vi "G#Object_GetAttributeValue.vi"(0 "reference in":refnum<class "G#Object.lvclass">, 1 "object attributes (T)":bool=TRUE, 2 "class attributes (F)":bool, 5 "error in (no error)":errorcluster) -> (14 "reference out":refnum<class "G#Object.lvclass">, 15 "attributes":variant[](array[variant]), 16 "class attributes":variant[](array[variant]), 17 "valid object":bool, 19 "error out":errorcluster)   [LabVIEW 2017, in "G#Object.lvclass"]
doc: "Returns the attribute values of all classes in the hierarchy that the object belongs to, represented as variants."
uses:
  G#Object.lvclass
  G#Object_State.ctl
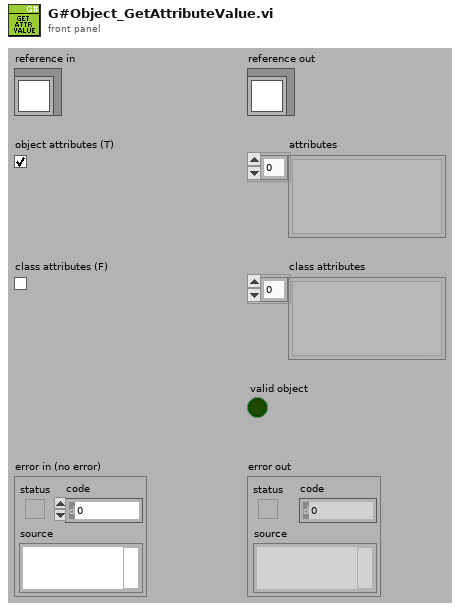
[diagram p1: front panel]
types:
  T1 = typedef "G#Object.lvclass/G#Object_State.ctl" = enum16{"Clear", "Create", "Delete", "Get class attributes", "Class hierarchy", "Get attribute value", "Set attribute value"}
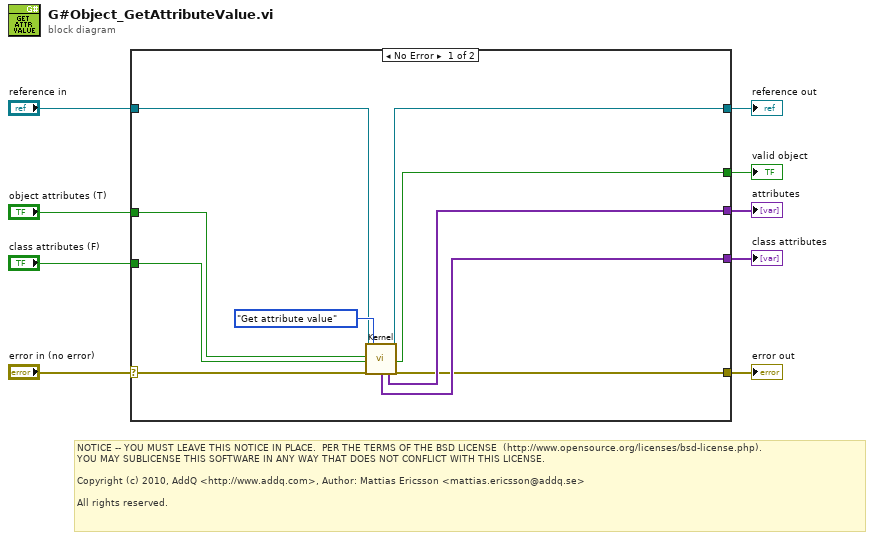
[diagram p0: block diagram]
diagram:
  # "NOTICE -- YOU MUST LEAVE THIS NOTICE IN PLACE.  PER THE TERMS OF THE BSD LICENSE  (http://www.opensource.org/licenses/bsd-license.php).\nYOU MAY SUBLICENSE THIS SOFTWARE IN ANY WAY THAT DOES NOT CONFLICT WITH THIS LICENSE.\n\nCopyright (c) 2010, AddQ <http://www.addq.com>, Author: Mattias Ericsson <mattias.ericsson@addq.se>\n\nAll rights reserved."
  n1 = case shown="No Error" "error in (no error)" {
    selector: "error in (no error)" -> [w13 w21]
    tunnel: [w12 w21] -> w8
    tunnel: [w10 w20] -> w6
    tunnel: "reference in" -> [w11 w20]
    tunnel: [w18 _] -> w5
    tunnel: [w17 _] -> w4
    tunnel: [w14 _] -> w3
    tunnel: "object attributes (T)" -> [w16 _]
    tunnel: "class attributes (F)" -> [w15 _]
    frame No Error {
      n2 = call-dynamic "Kernel.vi"("reference in"=w11, "option 1"=w16, "option 2"=w15, "error in (no error)"=w13, "state"=G#Object_State."Get attribute value" ("State")) -> ("class attributes out"=w17:variant[], "attributes out"=w18:variant[], "reference out"=w10:refnum<class "G#Object.lvclass">, "output 1"=w14:bool, "error out"=w12:errorcluster)  [unwired: 6 in, 4 out]
    }
    frame Error {
    }
  }
  "error out" <- w8
  "reference out" <- w6
  "attributes" <- w5
  "class attributes" <- w4
  "valid object" <- w3
